vi "build memory.vi"(8 "error in (no error)":errorcluster caption="에러 입력(에러 없음)", 10 "WF List":T1[](array[typedef]), 11 "DW7802 입력":refnum<class "DW7802.lvclass">) -> (0 "error out":errorcluster caption="에러 출력", 1 "memory data by wf":cluster{"Header":u8[], "Data":u8[]}[](array[cluster]), 2 "full memory data":u8[](array[numeric]), 3 "DW7802 출력":refnum<class "DW7802.lvclass">)   [LabVIEW 2020, in "DW7802.lvclass"]
uses:
  DW7802.lvclass
  SubVIs/Waveform Editor/Controls/(Ctrl)Waveform Editor_WF List.ctl
  Waveform Obj Class/Waveform Obj/Waveform Obj.lvclass
  Waveform Obj Class/Waveform Obj/Waveform Obj.lvclass/Waveform Obj.ctl
  Waveform Obj Class/Waveform Obj/Accessors/Read voltage range.vi
  Waveform Obj Class/Waveform Obj/Accessors/Read sampling rate.vi
  Waveform Obj Class/Waveform Obj/Accessors/Read play mode.vi
  DW7802.lvclass/DW7802.ctl
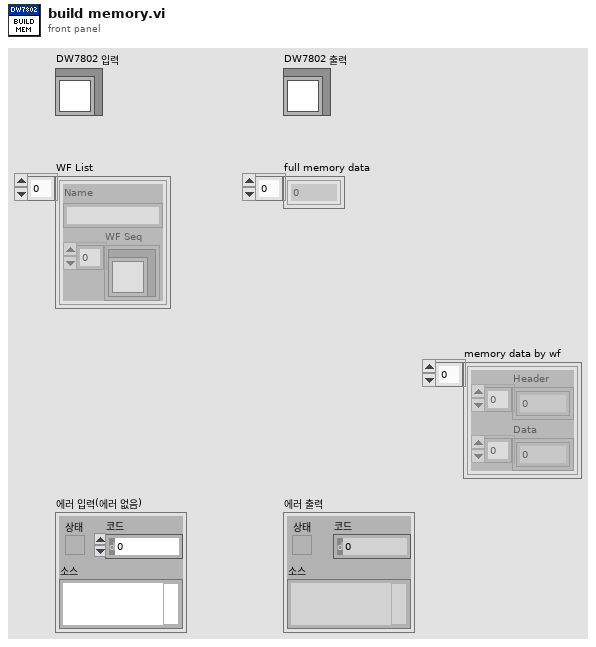
[diagram p1: front panel]
types:
  T1 = typedef "(Ctrl)Waveform Editor_WF List.ctl" = cluster{"Name":string, "WF Seq":refnum<class "Waveform Obj.lvclass">[]}
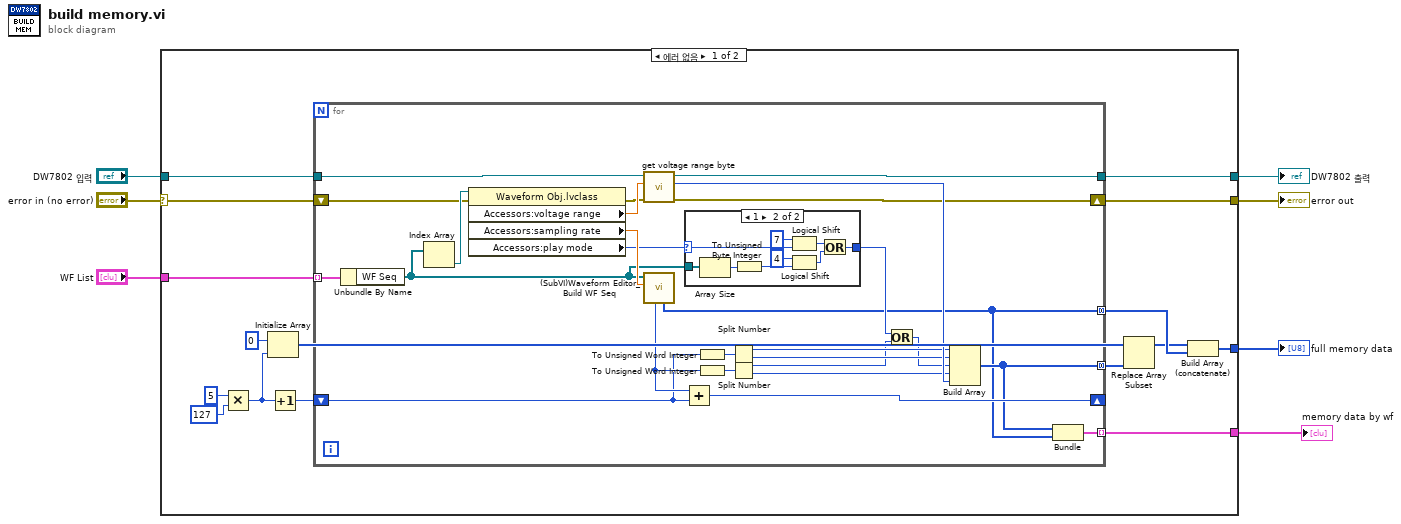
[diagram p0: block diagram]
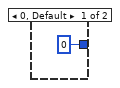
[diagram p2: hidden frame]
diagram:
  n1 = case shown="에러 없음" "error in (no error)" {
    selector: "error in (no error)" -> [w20 w60]
    tunnel: "DW7802 입력" -> [w21 w61]
    tunnel: "WF List" -> [w19 _]
    tunnel: [w18 w61] -> w6
    tunnel: [w17 w60] -> w4
    tunnel: [w16 _] -> w5
    tunnel: [w8 _] -> w1
    frame No Error {
      n2 = Multiply(x=5, y=127) -> (x*y=w12:i32)
      n3 = Initialize Array(u8 0 ("원소"), w12) -> (w10:u8[])
      n4 = Increment(x=w12) -> (x+1=w14:i32)
      n5 = for {
        tunnel: w19 -> [w48] mode=indexing
        shift-right: [w47] -> _
        shift-left: w14 -> [w24]
        tunnel: [w26] -> w22 mode=concatenating
        tunnel: w21 -> [w46]
        tunnel: [w27] -> w11 mode=concatenating
        tunnel: [w39] -> w18
        shift-right: [w38] -> w17
        shift-left: w20 -> [w35]
        tunnel: [w32] -> w8 mode=indexing
        n6 = Unbundle By Name(w48) -> ("WF Seq"=w29:refnum<class "Waveform Obj.lvclass">[])
        n7 = Index Array(array=w29) -> (element=w42:refnum<class "Waveform Obj.lvclass">)  [unwired: 1 in]
        n8 = property class="Waveform Obj.lvclass"(reference=w42, error in=w35) -> (error out=w34:errorcluster, "Accessors:voltage range"=w36:dbl, "Accessors:sampling rate"=w37:dbl, "Accessors:play mode"=w30:u8)  [unwired: 1 out]
        n9 = call-dynamic "get voltage range byte.vi"("error in (no error)"=w34, "voltage range"=w36, "DW7802 입력"=w46) -> ("error out"=w38:errorcluster, "byte value"=w49:u8, "DW7802 출력"=w39:refnum<class "DW7802.lvclass">)  [unwired: 6 in]
        n10 = call "(SubVI)Waveform Editor_Build WF Seq.vi"("Sampling Rate"=w37, "WF Seq"=w29) -> ("8bit memory data"=w26:u8[], "bytes of memory data"=w31:i32)  [unwired: 4 in, 4 out]
        n11 = Add(x=w31, y=w24) -> (x+y=w47:i32)
        n12 = case shown="1" w30 {
          selector: w30 -> [_ w57]
          tunnel: w29 -> [_ w59]
          tunnel: [u8 0 w51] -> w28
          frame 0, Default {
          }
          frame 1 {
            n13 = Array Size(array=w59) -> (size(s)=w58:i32)
            n14 = To Unsigned Byte Integer(number=w58) -> (unsigned 8bit integer=w55:u8)
            n15 = Logical Shift(y=i16 7, x=w57) -> (x << y=w53:u8)
            n16 = Logical Shift(y=i16 4, x=w55) -> (x << y=w52:u8)
            n17 = Or(x=w53, y=w52) -> (x .or. y?=w51:u8)
          }
        }
        n18 = To Unsigned Word Integer(number=w24) -> (unsigned 16bit integer=w44:u16)
        n19 = To Unsigned Word Integer(number=w31) -> (unsigned 16bit integer=w41:u16)
        n20 = Split Number(x=w44) -> (hi(x)=w45:u8, lo(x)=w43:u8)
        n21 = Split Number(x=w41) -> (hi(x)=w25:u8, lo(x)=w40:u8)
        n22 = Or(x=w28, y=w25) -> (x .or. y?=w33:u8)
        n23 = Build Array(w45, w43, w33, w40, w49) -> (w27:u8[])
        n24 = Bundle(w27, "8bit memory data"=w26) -> (w32:cluster{u8[], "8bit memory data":u8[]})  [unwired: 1 in]
      }
      n25 = Replace Array Subset(array=w10, new element=w11) -> (w9:u8[])  [unwired: 1 in]
      n26 = Build Array (concatenate)(w9, w22) -> (w16:u8[])
    }
    frame Error {
    }
  }
  "error out" <- w4
  "DW7802 출력" <- w6
  "full memory data" <- w5
  "memory data by wf" <- w1
